vi "toStringArray.vi"(8 "error in (no error)":errorcluster, 11 "RfRamp in":refnum<class "RfRamp.lvclass">) -> (0 "error out":errorcluster, 2 "eventStringArray":string[](array[string]), 3 "RfRamp out":refnum<class "RfRamp.lvclass">)   [LabVIEW 2011, in "Tools.lvlib" / "Scripting.lvlib" / "RfRamp.lvclass"]
uses:
  RfRamp.lvclass
  Rf Event/rf.lvclass
  RfRamp.lvclass/RfRamp.ctl
  ScriptEvent.lvclass
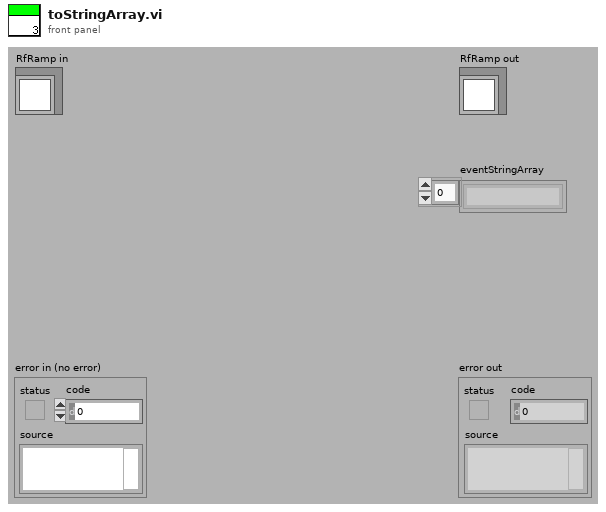
[diagram p1: front panel]
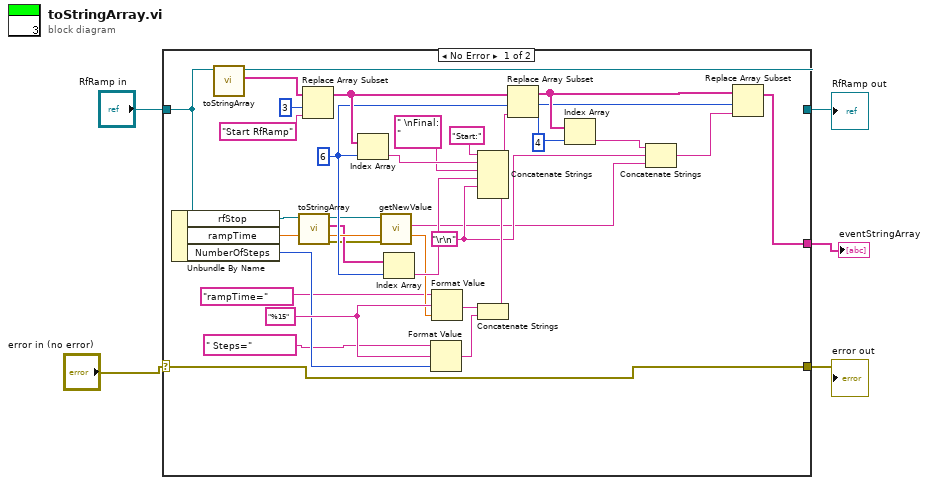
[diagram p0: block diagram]
diagram:
  n1 = case shown="No Error" "error in (no error)" {
    selector: "error in (no error)" -> [w37 w38]
    tunnel: [w37 w38] -> w4
    tunnel: [w26 w39] -> w3
    tunnel: "RfRamp in" -> [w36 w39]
    tunnel: [w10 _] -> w1
    frame No Error {
      w15 = 4
      w25 = "%15"
      w13 = "\r\n"
      w27 = 6
      n2 = Unbundle By Name(w36) -> ("rfStop"=w9:refnum<class "rf.lvclass">, "rampTime"=w23:dbl, "NumberOfSteps"=w22:i32)
      n3 = call-parent "toStringArray.vi"("rf in"=w36) -> ("eventStringArray"=w33:string[], "rf out"=w26:refnum<class "RfRamp.lvclass">)  [unwired: 8 in, 1 out]
      n4 = call-dynamic "toStringArray.vi"("rf in"=w9) -> ("error out"=w6:errorcluster, "eventStringArray"=w7:string[], "rf out"=w8:refnum<class "rf.lvclass">)  [unwired: 8 in]
      n5 = Replace Array Subset(array=w33, new element="Start RfRamp", index=3) -> (w29:string[])
      n6 = Index Array(array=w29, index=w27) -> (element=w32:string)
      n7 = call "getNewValue.vi"("error in (no error)"=w6, "ScriptEvent.lvclass in"=w8) -> ("newValue"=w12:string)  [unwired: 7 in, 2 out]
      n8 = Index Array(array=w7, index=w27) -> (element=w30:string)
      n9 = Format Value(string ("")=" Steps=", format string=w25, value (0)=w22) -> (output string=w24:string)
      n10 = Format Value(string ("")="rampTime=", format string=w25, value (0)=w23) -> (output string=w20:string)
      n11 = Concatenate Strings(w20, w24) -> (w19:string)
      n12 = Concatenate Strings("Start:", w32, " \nFinal: ", w30, w13, w19) -> (w28:string)
      n13 = Replace Array Subset(array=w29, new element=w28, index=w27) -> (w16:string[])
      n14 = Index Array(array=w16, index=w15) -> (element=w14:string)
      n15 = Concatenate Strings(w14, w13, w12) -> (w11:string)
      n16 = Replace Array Subset(array=w16, new element=w11, index=w15) -> (w10:string[])
    }
    frame Error {
    }
  }
  "error out" <- w4
  "RfRamp out" <- w3
  "eventStringArray" <- w1
